vi "Global rif vel freno.vi"() -> ()   [LabVIEW 2016]
panel:
  out "Rpm Rif vel freno":dbl
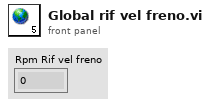
[diagram p1: front panel]
diagram:
